vi "Destroy.vi"(8 "error in (no error)":errorcluster, 11 "Image to File-Buffer Encoder in":refnum<class "Image to File-Buffer Encoder.lvclass">) -> (0 "error out":errorcluster)   [LabVIEW 2020, in "image.lvlib" / "Image to File-Buffer Encoder.lvclass"]
uses:
  Image to File-Buffer Encoder.lvclass
  Image to File-Buffer Encoder.lvclass/Image to File-Buffer Encoder.ctl
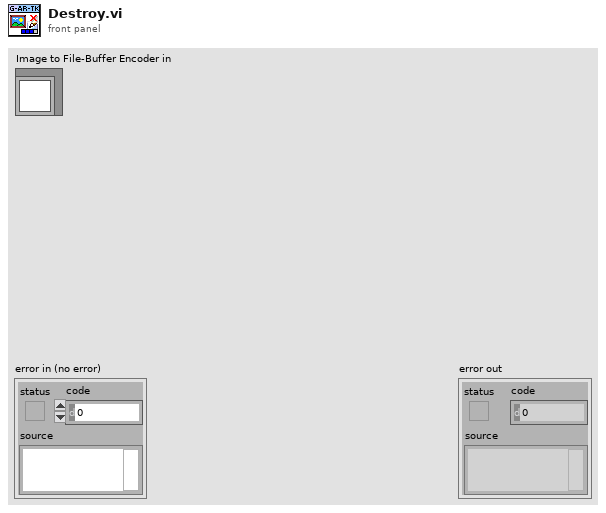
[diagram p1: front panel]
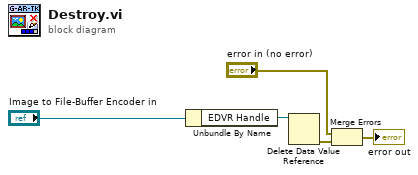
[diagram p0: block diagram]
diagram:
  n1 = Unbundle By Name("Image to File-Buffer Encoder in") -> ("EDVR Handle"=w3:refnum<data-value>)
  n2 = Delete Data Value Reference(data value reference=w3) -> (error out=w1:errorcluster)  [unwired: 1 in, 1 out]
  n3 = Merge Errors("error in (no error)", w1) -> (→"error out":errorcluster)
